vi "Objective scan with axial scan.vi"() -> ()   [LabVIEW 2020]
uses:
  <vilib>/DAQmx/write.llb/DAQmx Write (Analog 1D Wfm NChan NSamp).vi
  <vilib>/DAQmx/create/channels.llb/DAQmx Create Channel (AO-Voltage-Basic).vi
  <vilib>/DAQmx/configure/timing.llb/DAQmx Timing (Use Waveform).vi
  <vilib>/DAQmx/miscellaneous.llb/DAQmx Fill In Error Info.vi
  <vilib>/measure/NI_MABase.lvlib
panel:
  out "Camera trigger (red), Sawtooth input (blue) and Piezo trigger (green)":waveform(dbl)[](graph)=[{"t0"=timestamp(0 s since 1904-01-01), "dt"=0.001, "Y"=array[1000 elements]}, {"t0"=timestamp(0 s since 1904-01-01), "dt"=0.001, "Y"=array[1000 elements]}, {"t0"=timestamp(0 s since 1904-01-01), "dt"=0.001, "Y"=array[1000 elements]}]
  in  "Sawtooth Offset":dbl=0.025 format="%.2p"
  in  "Camera trigger delay (degrees)":dbl=-180.0 format="%.2p"
  in  "Exposure time (ms)":dbl=1000.0
  out "# Samples written per channel":u32=1000
  in  "Stop":bool
  in  "Sawtooth Phase":dbl=180.0 format="%.2p"
  in  "Sawtooth Amplitude":dbl=0.36 format="%.2p"
  # "Green ->piezo trigger\nRed ->camera trigger\n-2um step size, -100 steps \n500steps/sec, 10um/sec"
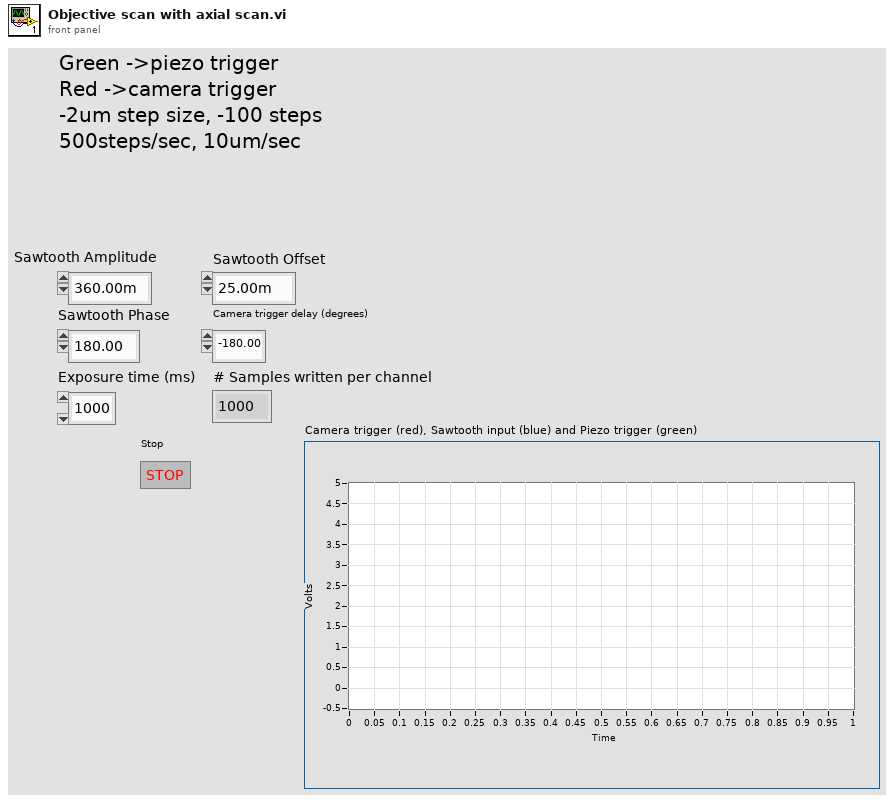
[diagram p1: front panel]
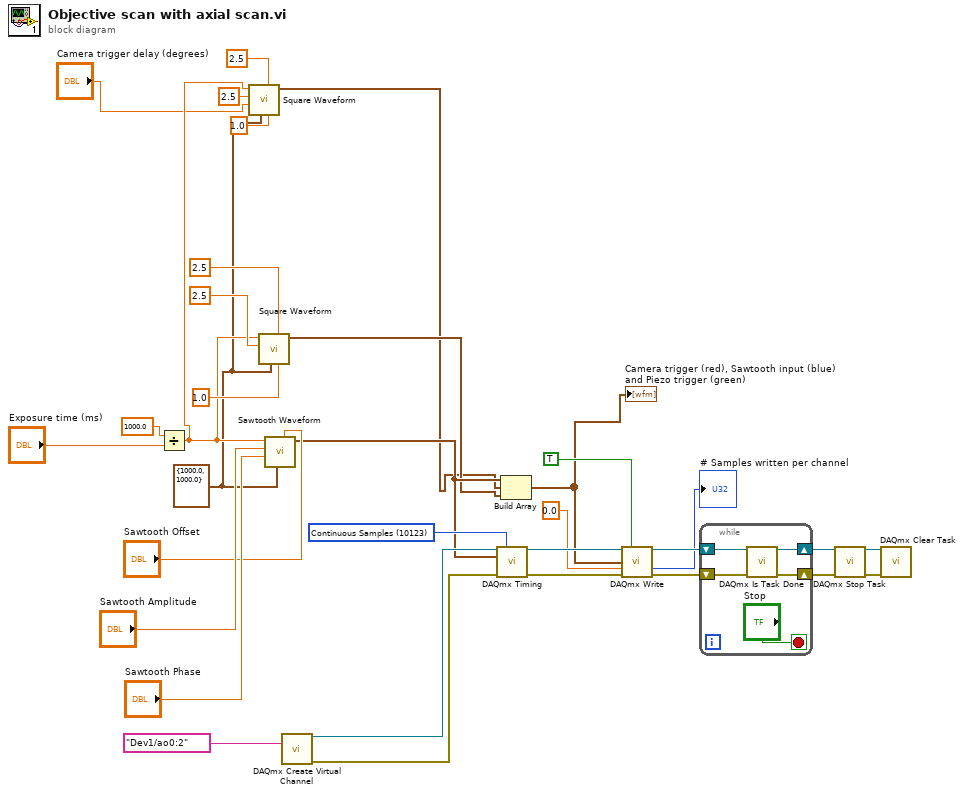
[diagram p0: block diagram]
diagram:
  w5 = cluster{"Fs":dbl, "#s":dbl} {"Fs"=1000.0, "#s"=1000.0} ("sampling info")
  w27 = 10123 items=["Finite Samples"=10178, "Continuous Samples"=10123, "Hardware Timed Single Point"=12522] ("sample mode")
  n1 = Divide(x=1000.0, y="Exposure time (ms)") -> (x/y=w7:dbl)
  n2 = call <vilib>:"Square Waveform.vi"("duty cycle (%)"=1.0, "offset"=2.5, "sampling info"=w5, "phase"="Camera trigger delay (degrees)", "amplitude"=2.5, "frequency"=w7) -> ("signal out"=w1:waveform(dbl))  [unwired: 4 in, 1 out]
  n3 = call <vilib>:"Square Waveform.vi"("duty cycle (%)"=1.0, "offset"=2.5, "sampling info"=w5, "amplitude"=2.5, "frequency"=w7) -> ("signal out"=w2:waveform(dbl))  [unwired: 5 in, 1 out]
  n4 = call <vilib>:"Sawtooth Waveform.vi"("offset"="Sawtooth Offset", "sampling info"=w5, "phase"="Sawtooth Phase", "amplitude"="Sawtooth Amplitude", "frequency"=w7) -> ("signal out"=w10:waveform(dbl))  [unwired: 5 in, 1 out]
  n5 = call-poly <vilib>:"DAQmx Create Virtual Channel.vi"("physical channels"=tag "Dev1/ao0:2") -> ("task out"=w29:refnum<k21>, "error out"=w28:errorcluster)  [unwired: 13 in]
  n6 = call-poly <vilib>:"DAQmx Timing.vi"("task/channels in"=w29, "sample mode"=w27, "waveform"=w10, "error in"=w28) -> ("task out"=w24:refnum<k21>, "error out"=w23:errorcluster)  [unwired: 10 in]
  n7 = Build Array(w10, w1, w2) -> (w3:waveform(dbl)[])
  "Camera trigger (red), Sawtooth input (blue) and Piezo trigger (green)" <- w3
  n8 = call-poly <vilib>:"DAQmx Write.vi"("task/channels in"=w24, "auto start"=TRUE, "data"=w3, "timeout"=0.0, "error in"=w23) -> ("task out"=w25:refnum<k21>, "number of samples written per channel"=→"# Samples written per channel":u32, "error out"=w26:errorcluster)  [unwired: 8 in]
  n9 = while {
    shift-right: [w35] -> w20
    shift-left: w25 -> [w38]
    shift-right: [w36] -> w21
    shift-left: w26 -> [w37]
    stop <- "Stop" stop-if-true
    n10 = call <vilib>:"DAQmx Is Task Done.vi"("task/channels in"=w38, "error in"=w37) -> ("task out"=w35:refnum<k21>, "error out"=w36:errorcluster)  [unwired: 11 in, 1 out]
  }
  n11 = call <vilib>:"DAQmx Stop Task.vi"("task/channels in"=w20, "error in"=w21) -> ("task out"=w30:refnum<k21>, "error out"=w31:errorcluster)  [unwired: 12 in]
  n12 = call <vilib>:"DAQmx Clear Task.vi"("task in"=w30, "error in"=w31) -> ()  [unwired: 13 in, 1 out]
